vi "GNSS RF Test Fetch Results.vi"(8 "error in (no error)":errorcluster, 11 "Template Tx Test in":refnum<class "niDTS GNSS RF Test.lvclass">) -> (0 "error out":errorcluster, 2 "Results":T1, 3 "Template Tx Test out":refnum<class "niDTS GNSS RF Test.lvclass">)   [LabVIEW 2015, in "niDTS GNSS.lvlib" / "niDTS GNSS RF Test.lvclass"]
uses:
  niDTS GNSS RF Test.lvclass
  Includes/niDTS GNSS RF Test INC Results.ctl
  Framework/Dut/Objects/BASE_class/niDTS Dut.lvclass
  niDTS GNSS.lvlib
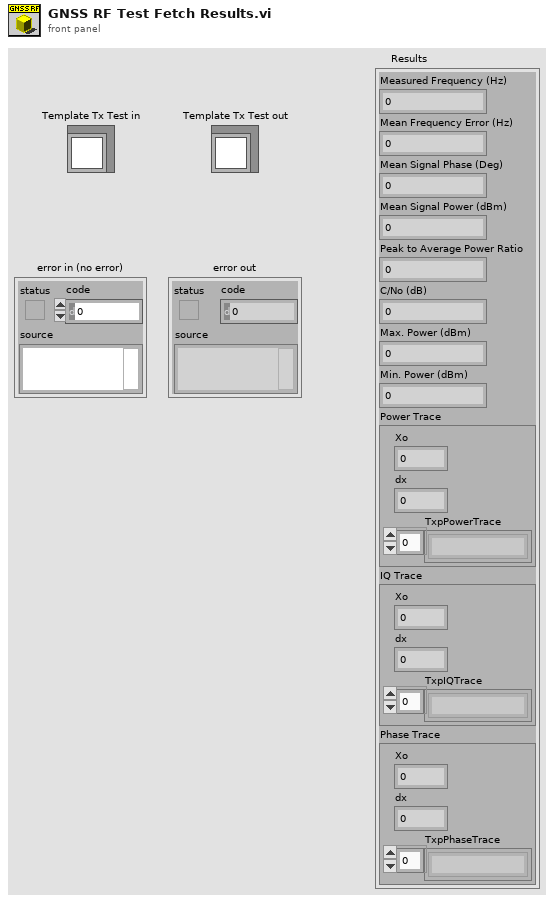
[diagram p1: front panel]
types:
  T1 = typedef "niDTS GNSS.lvlib/niDTS GNSS RF Test INC Results.ctl" = cluster{"Measured Frequency (Hz)":dbl, "Mean Frequency Error (Hz)":dbl, "Mean Signal Phase (Deg)":dbl, "Mean Signal Power (dBm)":dbl, "Peak to Average Power Ratio":dbl, "C/No (dB)":dbl, "Max. Power (dBm)":dbl, "Min. Power (dBm)":dbl, "Power Trace":cluster{"Xo":dbl, "dx":dbl, "TxpPowerTrace":string[]}, "IQ Trace":cluster{"Xo":dbl, "dx":dbl, "TxpIQTrace":string[]}, "Phase Trace":cluster{"Xo":dbl, "dx":dbl, "TxpPhaseTrace":string[]}}
  T2 = typedef "niDTS Framework.lvlib/niDTS Dut INC Handle.ctl" = refnum<data-value>
  T3 = cluster{"Xo":dbl, "dx":dbl, "TxpIQTrace":string[]}
  T4 = cluster{"Xo":dbl, "dx":dbl, "TxpPhaseTrace":string[]}
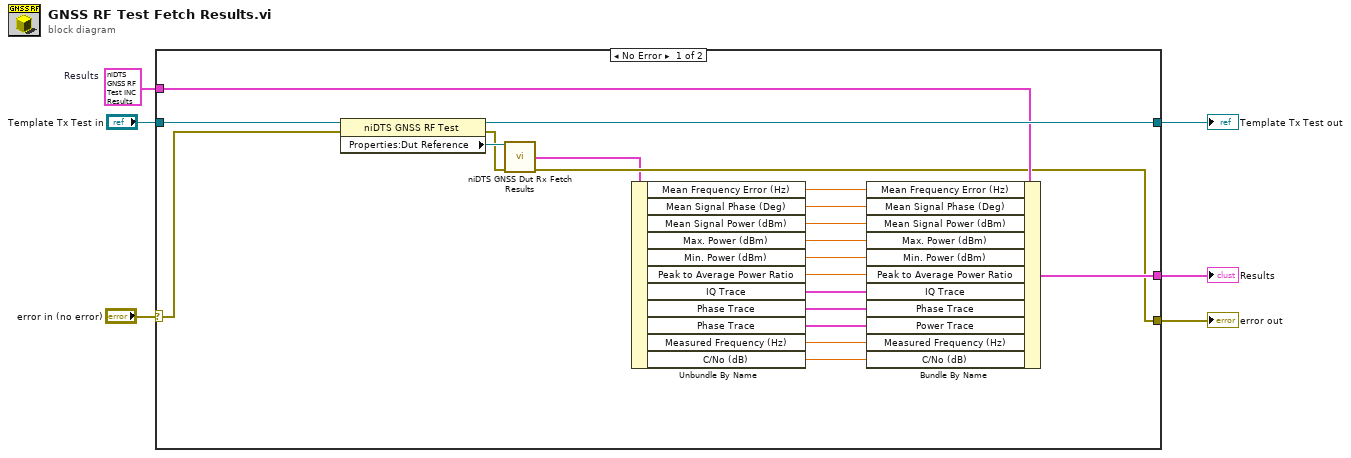
[diagram p0: block diagram]
diagram:
  w1 = T1 {"Measured Frequency (Hz)"=nan, "Mean Frequency Error (Hz)"=nan, "Mean Signal Phase (Deg)"=nan, "Mean Signal Power (dBm)"=nan, "Peak to Average Power Ratio"=nan, "C/No (dB)"=0.0, "Max. Power (dBm)"=nan, "Min. Power (dBm)"=nan, "Power Trace"={"Xo"=nan, "dx"=nan, "TxpPowerTrace"=[]}, "IQ Trace"={"Xo"=nan, "dx"=nan, "TxpIQTrace"=[]}, "Phase Trace"={"Xo"=nan, "dx"=nan, "TxpPhaseTrace"=[]}}  # Results
  n1 = case shown="No Error" "error in (no error)" {
    selector: "error in (no error)" -> [w25 w29]
    tunnel: [w19 w29] -> w5
    tunnel: [w24 w28] -> w3
    tunnel: "Template Tx Test in" -> [w23 w28]
    tunnel: [w26 w27] -> w2
    tunnel: w1 -> [w22 w27]
    frame No Error {
      n2 = property class="niDTS GNSS RF Test"(reference=w23, error in=w25) -> (reference out=w24:refnum<class "niDTS GNSS RF Test.lvclass">, error out=w20:errorcluster, "Properties:Dut Reference"=w21:T2)
      n3 = call "niDTS GNSS Dut Rx Fetch Results.vi"("Dut Handle in"=w21, "error in (no error)"=w20) -> ("Results"=w18:T1, "error out"=w19:errorcluster)  [unwired: 11 in, 1 out]
      n4 = Unbundle By Name(w18) -> ("Mean Frequency Error (Hz)"=w17:dbl, "Mean Signal Phase (Deg)"=w16:dbl, "Mean Signal Power (dBm)"=w15:dbl, "Max. Power (dBm)"=w14:dbl, "Min. Power (dBm)"=w13:dbl, "Peak to Average Power Ratio"=w12:dbl, "IQ Trace"=w11:T3, "Phase Trace"=w10:T4, "Phase Trace"=w9:T4, "Measured Frequency (Hz)"=w8:dbl, "C/No (dB)"=w7:dbl)
      n5 = Bundle By Name(cluster=w22, "Mean Frequency Error (Hz)"=w17, "Mean Signal Phase (Deg)"=w16, "Mean Signal Power (dBm)"=w15, "Max. Power (dBm)"=w14, "Min. Power (dBm)"=w13, "Peak to Average Power Ratio"=w12, "IQ Trace"=w11, "Phase Trace"=w10, "Power Trace"=w9, "Measured Frequency (Hz)"=w8, "C/No (dB)"=w7) -> (w26:T1)
    }
    frame Error {
    }
  }
  "error out" <- w5
  "Template Tx Test out" <- w3
  "Results" <- w2
